vi "9_20_Fxp_addation.vi"(1 "y":fxp<+/-,20,9>, 2 "x":fxp<+/-,20,9>) -> (0 "x+y":fxp<+/-,21,10> format="%.41g")   [LabVIEW 2020]
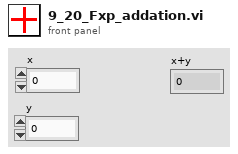
[diagram p1: front panel]
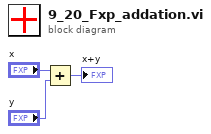
[diagram p0: block diagram]
diagram:
  n1 = Add(x="x", y="y") -> (x+y=→"x+y":fxp<+/-,21,10>)
